vi "USRP Packet Transmitter.vi"() -> ()   [LabVIEW 2013]
uses:
  <vilib>/addons/Modulation/niDMT.lvlib
  <vilib>/addons/Modulation/Digital/General/MT Generate PSK System Parameters(M).vi
  <instrlib>/niUSRP/niUSRP Write Tx Data (CDB Cluster).vi
panel:
  in  "autoscale":bool
  out "Constellation Graph":T1(graph)
  out "Symbol Rate\n[symbols/sec]":dbl=50000.0 format="%#.6p"
  in  "stop":bool
  in  "Tab Control":T2(tab)=enum."Tx Parameters"
  in  "Message Text":string="Two roads diverged in a yellow wood,\nAnd sorry I could not travel both\nAnd be one traveler, long I stood\nAnd looked down one as far as I could\nTo where it bent in the undergrowth.\n\nThen took the other, as just as fair,\nAnd having perhaps the better claim,\nBecause it was grassy and wanted wear;\nThough as for that the passing there\nHad worn them really about the same.\n\nAnd both that morning equally lay\nIn leaves no step had trodden black.\nOh, I kept the first for another day!\nYet knowing how way leads on to way,\nI doubted if I should ever come back.\n\nI shall be telling this with a sigh\nSomewhere ages and ages hence:\nTwo roads diverged in a wood, and I--\nI took the one less traveled by,\nAnd that has made all the difference.\n"
  in  "Message Type":bool=TRUE
  in  "Packet Parameters":T3={"Guard Bits "=30, "Sync Bits"=20, "Message Bits"=128}
  in  "Packet Pad \n[samples]":i32=200
  in  "Blank Frame \n[samples]":i32=500
  out "Number of Packets in Message":i32=46
  in  "PN sequence order\nfor Sync Bits":i32=31 caption="PN sequence order (9)"
  in  "Select PSK Modulation Format":T4(tab)=enum."QPSK" caption="PSK"
  in  "BPSK System Parameters":T5={"Samples per Symbol"=8, "symbol map"=[], "Differential PSK"=enum."disable", "PSK type"=0} {"PSK type" items=["normal", "shifted", "offset"]; "symbol map" format="%.3f"}
  in  "QPSK System Parameters":T5={"Samples per Symbol"=8, "symbol map"=[], "Differential PSK"=enum."disable", "PSK type"=0} {"PSK type" items=["normal", "shifted", "offset"]; "symbol map" format="%.3f"}
  in  "pi/4 DQPSK System Parameters":T5={"Samples per Symbol"=8, "symbol map"=[], "Differential PSK"=enum."enable", "PSK type"=1} {"PSK type" items=["normal", "shifted", "offset"]; "symbol map" format="%.3f"}
  in  "OQPSK System Parameters":T5={"Samples per Symbol"=8, "symbol map"=[], "Differential PSK"=enum."disable", "PSK type"=2} {"PSK type" items=["normal", "shifted", "offset"]; "symbol map" format="%.3f"}
  in  "8-PSK System Parameters":T5={"Samples per Symbol"=8, "symbol map"=[], "Differential PSK"=enum."disable", "PSK type"=0} {"PSK type" items=["normal", "shifted", "offset"]; "symbol map" format="%.3f"}
  in  "16-PSK System Parameters":T5={"Samples per Symbol"=8, "symbol map"=[], "Differential PSK"=enum."disable", "PSK type"=0} {"PSK type" items=["normal", "shifted", "offset"]; "symbol map" format="%.3f"}
  in  "M":i32=4 min=2 step=2
  in  "Custom System Parameters":T5={"Samples per Symbol"=8, "symbol map"=[], "Differential PSK"=enum."disable", "PSK type"=0} {"PSK type" items=["normal", "shifted", "offset"]; "symbol map" format="%.3f"}
  in  "Pulse Shaping Filter Parameters":T6={"Alpha"=0.5, "Filter Length"=6, "TX Filter"=enum."Root Raised Cos"} caption="Pulse Shaping Filter" {"Alpha" format="%.2f"}
  in  "Tx Parameters":T7={"Tx IQ Sampling\nRate [s/sec]"=400000.0, "Tx Frequency [Hz]"=915000000.0, "Tx Gain [dB]"=0.0, "Tx Antenna"="TX1"} {"Tx Gain [dB]" format="%#.6p"; "Tx Frequency [Hz]" format="%#.6p"; "Tx IQ Sampling\nRate [s/sec]" format="%#.6p"}
  out "Actual Tx Parameters":T7={"Tx IQ Sampling\nRate [s/sec]"=400000.0, "Tx Frequency [Hz]"=915000000.0, "Tx Gain [dB]"=0.0, "Tx Antenna"="TX1"} {"Tx Gain [dB]" format="%#.6p"; "Tx Frequency [Hz]" format="%#.6p"; "Tx IQ Sampling\nRate [s/sec]" format="%#.6p"}
  in  "USRP IP address":refnum<k15>="192.168.10.2"
  out "error out":errorcluster
  in  "Queue Length":i32=10
  # "Packet Transmitter"
  # "Custom Text"
  # "PN Sequence"
  # "Guard\nBand"
  # "Sync\nSeq"
  # "Packet\nNumber"
  # "Pad\nData"
  # "Blank\nFrame"
  # "Data"
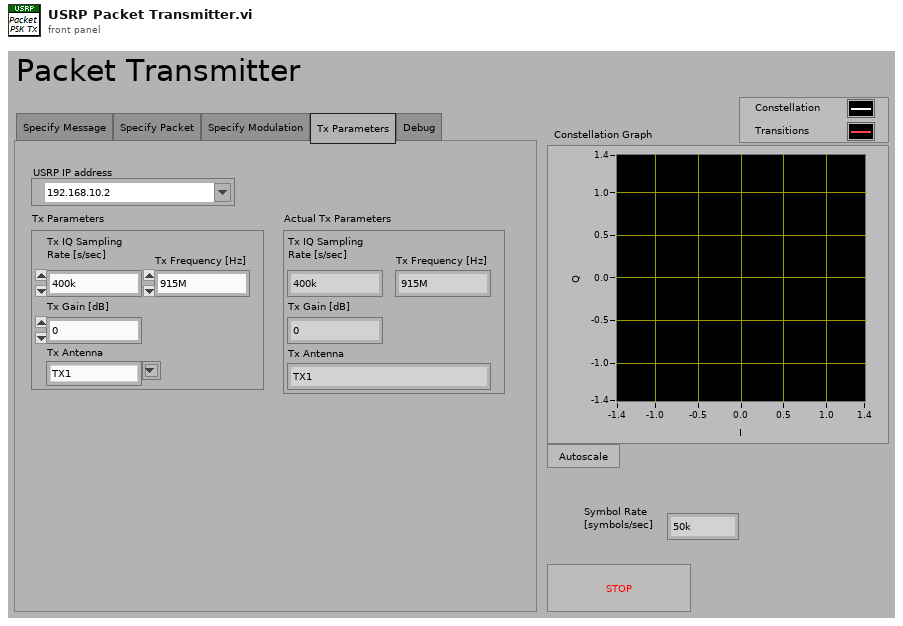
[diagram p1: front panel]
types:
  T1 = cluster{"Decimated Array":dbl[], "Decimated Array":dbl[]}[]
  T2 = enum32{"Specify Message", "Specify Packet", "Specify Modulation", "Tx Parameters", "Debug"}
  T3 = cluster{"Guard Bits ":i32, "Sync Bits":i32, "Message Bits":i32}
  T4 = enum32{"BPSK", "QPSK", "pi/4DQPSK", "OQPSK", "8-PSK", "16-PSK", "Custom"}
  T5 = cluster{"Samples per Symbol":i32, "symbol map":cdb[], "Differential PSK":enum16{"disable", "enable"}, "PSK type":u16}
  T6 = cluster{"Alpha":dbl, "Filter Length":i32, "TX Filter":enum16{"none", "Raised Cosine", "Root Raised Cos", "Gaussian"}}
  T7 = cluster{"Tx IQ Sampling\nRate [s/sec]":dbl, "Tx Frequency [Hz]":dbl, "Tx Gain [dB]":dbl, "Tx Antenna":string}
  T8 = cluster{"samples per symbol (16)":i32, "symbol map":cdb[], "differential PSK":enum16{"disable", "enable"}, "PSK type":u16}
  T9 = cluster{"s? t:f":cluster{"t0":dbl, "dt":dbl, "Y":cdb[]}, i32}
  T10 = cluster{"output complex waveform":cluster{"t0":dbl, "dt":dbl, "Y":cdb[]}, i32}
  T11 = cluster{"constellation":dbl[], "oversampled data":dbl[]}[]
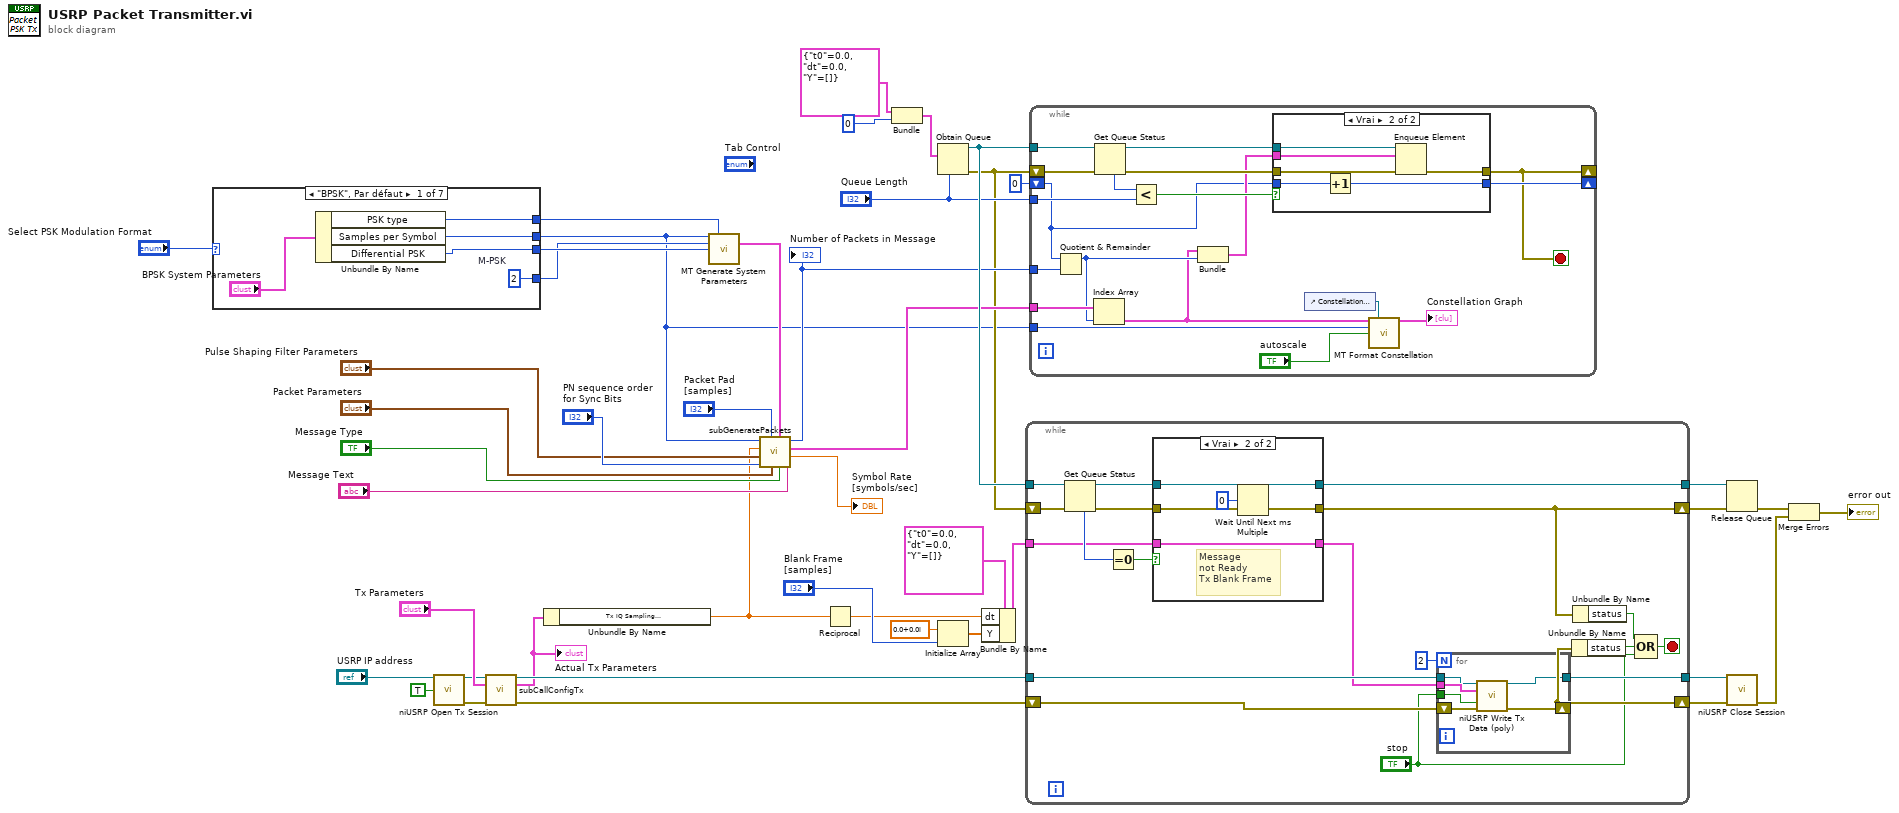
[diagram p0: block diagram]
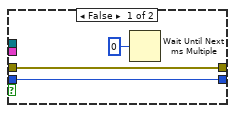
[diagram p2: hidden frame]
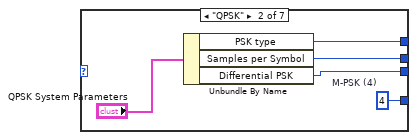
[diagram p3: hidden frame]
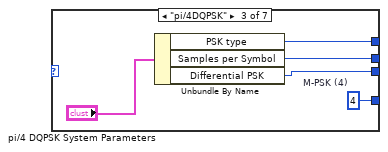
[diagram p4: hidden frame]
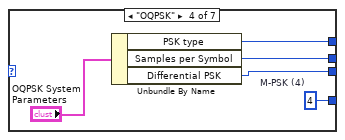
[diagram p5: hidden frame]
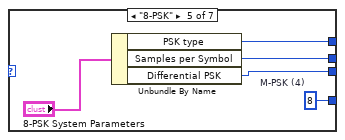
[diagram p6: hidden frame]
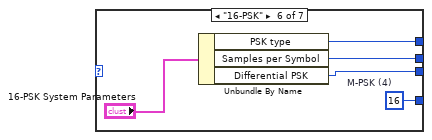
[diagram p7: hidden frame]
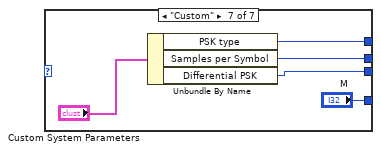
[diagram p8: hidden frame]
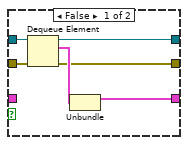
[diagram p9: hidden frame]
diagram:
  n1 = case shown="\"BPSK\", Par défaut" "Select PSK Modulation Format" {
    tunnel: [w46 w50 w58 w63 w68 w74 w77] -> w2
    tunnel: [w47 w52 w57 w62 w67 w73 w78] -> w43
    tunnel: [w49 w54 w59 w64 w66 w72 "M"] -> w24
    tunnel: [w48 w53 w56 w61 w69 w71 w79] -> w11
    frame "BPSK", Default {
      w49 = 2  # M-PSK
      n2 = Unbundle By Name("BPSK System Parameters") -> ("PSK type"=w48:u16, "Samples per Symbol"=w46:i32, "Differential PSK"=w47:enum16{"disable", "enable"})
    }
    frame "QPSK" {
      w54 = 4  # M-PSK (4)
      n3 = Unbundle By Name("QPSK System Parameters") -> ("PSK type"=w53:u16, "Samples per Symbol"=w50:i32, "Differential PSK"=w52:enum16{"disable", "enable"})
    }
    frame "pi/4DQPSK" {
      w59 = 4  # M-PSK (4)
      n4 = Unbundle By Name("pi/4 DQPSK System Parameters") -> ("PSK type"=w56:u16, "Samples per Symbol"=w58:i32, "Differential PSK"=w57:enum16{"disable", "enable"})
    }
    frame "OQPSK" {
      w64 = 4  # M-PSK (4)
      n5 = Unbundle By Name("OQPSK System Parameters") -> ("PSK type"=w61:u16, "Samples per Symbol"=w63:i32, "Differential PSK"=w62:enum16{"disable", "enable"})
    }
    frame "8-PSK" {
      w66 = 8  # M-PSK (4)
      n6 = Unbundle By Name("8-PSK System Parameters") -> ("PSK type"=w69:u16, "Samples per Symbol"=w68:i32, "Differential PSK"=w67:enum16{"disable", "enable"})
    }
    frame "16-PSK" {
      w72 = 16  # M-PSK (4)
      n7 = Unbundle By Name("16-PSK System Parameters") -> ("PSK type"=w71:u16, "Samples per Symbol"=w74:i32, "Differential PSK"=w73:enum16{"disable", "enable"})
    }
    frame "Custom" {
      n8 = Unbundle By Name("Custom System Parameters") -> ("PSK type"=w79:u16, "Samples per Symbol"=w77:i32, "Differential PSK"=w78:enum16{"disable", "enable"})
    }
  }
  n9 = call <instrlib>:"niUSRP Open Tx Session.vi"("device names"="USRP IP address", "reset"=TRUE) -> ("session handle out"=w15:refnum<k15>, "error out"=w14:errorcluster)  [unwired: 12 in]
  n10 = call "subCallConfigTx.vi"("session handle"=w15, "Tx Parameters"="Tx Parameters", "error in"=w14) -> ("session handle out"=w23:refnum<k15>, "Actual Tx Parameters"=w22:T7, "error out"=w29:errorcluster)  [unwired: 10 in]
  "Actual Tx Parameters" <- w22
  n11 = Unbundle By Name(w22) -> ("Tx IQ Sampling\nRate [s/sec]"=w3:dbl)
  n12 = call-poly <vilib>:"MT Generate System Parameters.vi"("samples per symbol (16)"=w2, "PSK type"=w11, "M-PSK (4)"=w24, "differential PSK"=w43) -> ("PSK system parameters"=w12:T8)  [unwired: 9 in, 2 out]
  n13 = call "subGeneratePackets.vi"("Message Text"="Message Text", "Message Type"="Message Type", "PSK system parameters"=w12, "Packet Parameters"="Packet Parameters", "Packet Pad \n[samples]"="Packet Pad \n[samples]", "PN sequence order\nfor Sync Bits"="PN sequence order\nfor Sync Bits", "Pulse Shaping Filter Parameters"="Pulse Shaping Filter Parameters", "Tx IQ Sampling\nRate [s/sec]"=w3, "Samples per Symbol"=w2) -> ("Symbol Rate"=→"Symbol Rate\n[symbols/sec]":dbl, "Packets"=w31:cluster{"t0":dbl, "dt":dbl, "Y":cdb[]}[], "Number of Packets"=w21:i32)
  "Number of Packets in Message" <- w21
  n14 = Reciprocal(x=w3) -> (1/x=w25:dbl)
  n15 = Bundle("s? t:f"=cluster{"t0":dbl, "dt":dbl, "Y":cdb[]} {"t0"=0.0, "dt"=0.0, "Y"=[]}, 0) -> (w34:T9)  [unwired: 1 in]
  n16 = Obtain Queue(max queue size (-1, unlimited)="Queue Length", element data type=w34) -> (queue out=w40:refnum<queue>, error out=w17:errorcluster)  [unwired: 3 in, 1 out]
  n17 = Initialize Array(cdb 0.0+0.0i ("element"), "Blank Frame \n[samples]") -> (w39:cdb[])
  n18 = Bundle By Name(cluster=cluster{"t0":dbl, "dt":dbl, "Y":cdb[]} {"t0"=0.0, "dt"=0.0, "Y"=[]} ("s? t:f"), "dt"=w25, "Y"=w39) -> (w38:cluster{"t0":dbl, "dt":dbl, "Y":cdb[]})
  n19 = while {
    tunnel: w23 -> [w89]
    shift-right: [w86] -> w28
    shift-left: w29 -> [w90]
    tunnel: w40 -> [w98]
    tunnel: w38 -> [w95]
    tunnel: [w94] -> w37
    tunnel: [w88] -> w27
    shift-right: [w82] -> w36
    shift-left: w17 -> [w91]
    stop <- w85 stop-if-true
    n20 = Get Queue Status(queue=w98, error in (no error)=w91) -> (queue out=w93:refnum<queue>, error out=w92:errorcluster, # elements in queue=w97:i32)  [unwired: 1 in, 5 out]
    n21 = Equal To 0?(x=w97) -> (x = 0?=w96:bool)
    n22 = case shown="Vrai" w96 {
      tunnel: w95 -> [_ w114]
      tunnel: [w106 w114] -> w80
      tunnel: [w110 w112] -> w94
      tunnel: [w105 w113] -> w82
      tunnel: w93 -> [w109 w112]
      tunnel: w92 -> [w108 w113]
      frame False {
        n23 = Dequeue Element(queue=w109, error in (no error)=w108) -> (queue out=w110:refnum<queue>, element=w107:T9, error out=w105:errorcluster)  [unwired: 1 in, 1 out]
        n24 = Unbundle(w107) -> ("s? t:f"=w106:cluster{"t0":dbl, "dt":dbl, "Y":cdb[]})  [unwired: 1 out]
      }
      frame True {
        # "Message\nnot Ready\nTx Blank Frame"
        n25 = Wait Until Next ms Multiple(millisecond multiple=u32 0) -> ()  [unwired: 1 out]
      }
    }
    n26 = for {
      N: 2 -> [_]
      tunnel: w80 -> [w103]
      tunnel: w89 -> [w102]
      tunnel: [w101] -> w88
      tunnel: "stop" -> [w100]
      shift-right: [w99] -> w86
      shift-left: w90 -> [w104]
      n27 = call-poly <instrlib>:"niUSRP Write Tx Data (poly).vi"("session handle"=w102, "data"=w103, "end of data?"=w100, "error in (no error)"=w104) -> ("session handle out"=w101:refnum<k15>, "error out"=w99:errorcluster)  [unwired: 10 in]
    }
    n28 = Unbundle By Name(w86) -> ("status"=w87:bool)
    n29 = Unbundle By Name(w82) -> ("status"=w81:bool)
    n30 = Compound Arithmetic op=OR(w81, w87, "stop") -> (w85:bool)
  }
  n31 = while {
    tunnel: w40 -> [w133]
    shift-right: [w126] -> _
    shift-left: 0 -> [w122]
    tunnel: w31 -> [w123]
    tunnel: "Queue Length" -> [w125]
    tunnel: w21 -> [w124]
    shift-right: [w120] -> _
    shift-left: w17 -> [w128]
    tunnel: w2 -> [w117]
    stop <- w120 stop-if-true
    n32 = Quotient & Remainder(x=w122, y=w124) -> (x-y*floor(x/y)=w121:i32)  [unwired: 1 out]
    n33 = Index Array(array=w123, index=w121) -> (element=w115:cluster{"t0":dbl, "dt":dbl, "Y":cdb[]})
    n34 = Get Queue Status(queue=w133, error in (no error)=w128) -> (queue out=w132:refnum<queue>, error out=w129:errorcluster, # elements in queue=w131:i32)  [unwired: 1 in, 5 out]
    n35 = Less?(x=w131, y=w125) -> (x < y?=w130:bool)
    n36 = Bundle("output complex waveform"=w115, w121) -> (w127:T10)  [unwired: 1 in]
    n37 = case shown="Vrai" w130 {
      tunnel: w129 -> [w134 w142]
      tunnel: w132 -> [_ w141]
      tunnel: [w134 w140] -> w120
      tunnel: w127 -> [_ w139]
      tunnel: w122 -> [w136 w138]
      tunnel: [w136 w137] -> w126
      frame False {
        n38 = Wait Until Next ms Multiple(millisecond multiple=u32 0) -> ()  [unwired: 1 out]
      }
      frame True {
        n39 = Increment(x=w138) -> (x+1=w137:i32)
        n40 = Enqueue Element(queue=w141, element=w139, error in (no error)=w142) -> (error out=w140:errorcluster)  [unwired: 1 in, 2 out]
      }
    }
    n41 = control-ref of="Constellation Graph"() -> (w118:refnum<vi>)
    n42 = call <vilib>:"MT Format Constellation.vi"("waveform"=w115, "constellation reference"=w118, "samples per symbol"=w117, "autoscale"="autoscale") -> ("constellation graph"=→"Constellation Graph":T11)  [unwired: 1 in, 10 out]
  }
  n43 = Release Queue(queue=w37, error in (no error)=w36) -> (error out=w10:errorcluster)  [unwired: 3 out]
  n44 = call <instrlib>:"niUSRP Close Session.vi"("session handle"=w27, "error in (no error)"=w28) -> ("error out"=w9:errorcluster)  [unwired: 13 in]
  n45 = Merge Errors(w10, w9) -> (→"error out":errorcluster)
